vi "Send Command.vi"(6 "Timeout":i32, 7 "Message Transport":refnum<class "Message Transport Interface.lvclass">, 8 "error in (no error)":errorcluster, 9 "Message Priority":T1, 10 "Command Message":refnum<class "Command Message Interface.lvclass">, 11 "Mediated Actor in":refnum<class "Mediated Actor.lvclass">) -> (0 "error out":errorcluster, 3 "Mediated Actor out":refnum<class "Mediated Actor.lvclass">)   [LabVIEW 2016, in "Stream Mediator.lvlib" / "Mediated Actor.lvclass"]
doc: "--\nCopyright © 2017 Composed SystemsI All rights reserved.\n\nAuthor: Jon McBee <jon.mcbee@composed.io>\n\nThis library is provided \"AS IS\" ,WITHOUT WARRANTIES OR\nCONDITIONS OF ANY KIND, either express or implied.\n\nComposed Systems -- composed.io\n\nStream 0.0.1.1\nJon McBee - Composed Systems\nCopyright (c) 2017, Composed Systems"
uses:
  <userlib>/Composed Systems/Stream/Mediator/Classes/Mediated Actor/Mediated Actor.lvclass
  C:/Program Files (x86)/National Instruments/LabVIEW 2016/user.lib/Composed Systems/Stream/Actor/Actor Class/Ancestral Actor.lvclass
  <userlib>/Composed Systems/Stream/Mediator/Classes/Message Command Interface/Command Message Interface.lvclass
  C:/Program Files (x86)/National Instruments/LabVIEW 2016/user.lib/Composed Systems/Stream/Mediator/Classes/Message Interface/Message Interface.lvclass
  <userlib>/Composed Systems/Stream/Mediator/Classes/Message Transport Interface/Message Transport Interface.lvclass
  <userlib>/Composed Systems/Stream/Mediator/Classes/Message Transport Interface/Message Priority.ctl
  <userlib>/Composed Systems/Stream/Actor/Actor Class/Ancestral Actor.lvclass/Ancestral Actor.ctl
  <userlib>/Composed Systems/Stream/Mediator/Classes/Message Command Interface/Command Message Interface.lvclass/Command Message Interface.ctl
  <userlib>/Composed Systems/Stream/Actor/Actor Class/Ancestral Actor.lvclass
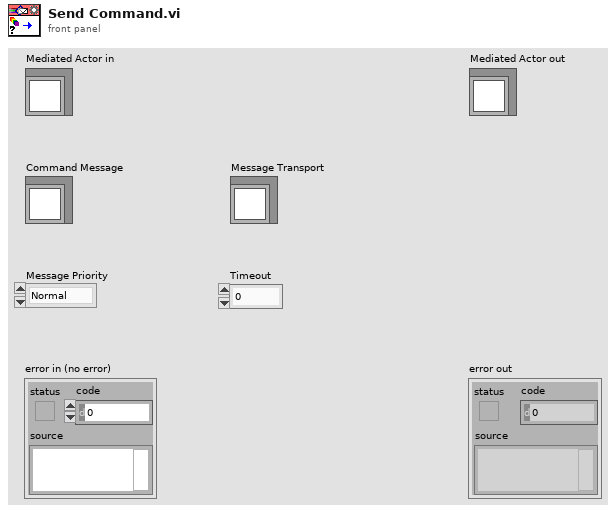
[diagram p1: front panel]
types:
  T1 = typedef "Stream Mediator.lvlib/Message Transport Interface.lvclass/Message Priority.ctl" = enum16{"Normal", "High"}
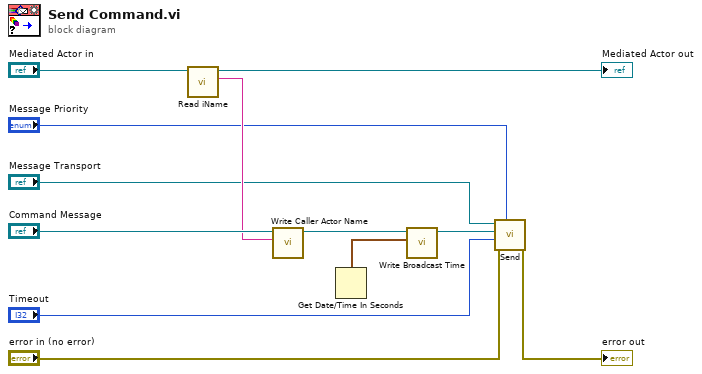
[diagram p0: block diagram]
diagram:
  n1 = call <userlib>:"Read iName.vi"("Ancestral Actor in"="Mediated Actor in") -> ("iName"=w8:string, "Ancestral Actor out"=→"Mediated Actor out":refnum<class "Mediated Actor.lvclass">)  [unwired: 8 in, 1 out]
  n2 = call <userlib>:"Write Caller Actor Name.vi"("Caller Actor Name"=w8, "Command Message Interface in"="Command Message") -> ("Command Message Interface out"=w9:refnum<class "Command Message Interface.lvclass">)  [unwired: 9 in]
  n3 = Get Date/Time In Seconds() -> (seconds since 1Jan1904=w7:timestamp)
  n4 = call <userlib>:"Write Broadcast Time.vi"("Broadcast Time"=w7, "Command Message Interface in"=w9) -> ("Command Message Interface out"=w6:refnum<class "Command Message Interface.lvclass">)  [unwired: 9 in]
  n5 = call-dynamic "Send.vi"("Message Priority"="Message Priority", "error in (no error)"="error in (no error)", "Timeout"="Timeout", "Message"=w6, "Message Transport Interface in"="Message Transport") -> ("error out"=→"error out":errorcluster)  [unwired: 4 in, 2 out]
